vi "SetAllPulsersGUI.vi"(7 "Init Tabor?":bool=TRUE, 8 "Tabor handle in":refnum<k15>, 11 "Pulser":T1) -> ()   [LabVIEW 2022 SP3]
uses:
  pulser.ctl
  PulserGlobals.vi
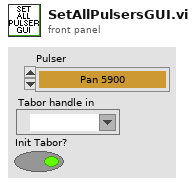
[diagram p1: front panel]
types:
  T1 = typedef "pulser.ctl" = enum16{"Pan 5900", "Daxsonics", "Agilent 33xxx", "UTEX", "JSR", "WMC Mono-Cycle", "No Pulser", "NYU AVTECH", "Tabor W1281A", "Pan 5800", "Unlisted", "Tabor WX2182B"}
  T2 = typedef "Daxsonics_Pulsers.ctl" = enum16{"BP1", "BP2_A", "BP2_B", "10ERS8", "New2021"}
  T3 = typedef "JSR Complete.ctl" = cluster{"JSR Pulse Settings":T4, "JSR Receive Settings":T9, "JSR Trigger Settings":T14}
  T4 = typedef "JSR Pulse.ctl" = cluster{"Damping":T5, "Pulse Energy Level":T6, "Pulser Impedance":T7, "Pulser Voltage (V)":T8}
  T5 = typedef "Damping.ctl" = i16
  T6 = typedef "Energy.ctl" = u16
  T7 = typedef "Z.ctl" = u16
  T8 = typedef "Volt.ctl" = i16
  T9 = typedef "JSR Recieve.ctl" = cluster{"Receiver Mode":T10, "High Pass Filter":T11, "Low Pass Filter":T12, "Gain (dB)":T13}
  T10 = typedef "Mode.ctl" = i8
  T11 = typedef "HPF.ctl" = u16
  T12 = typedef "LPF.ctl" = u16
  T13 = typedef "Gain.ctl" = i8
  T14 = typedef "JSR Trigger.ctl" = cluster{"External Trigger Limit":T15, "Trigger Source":T16, "PRF (Hz)":T17}
  T15 = typedef "Trig Limit.ctl" = i8
  T16 = typedef "Trig Source.ctl" = i8
  T17 = typedef "PRF.ctl" = dbl
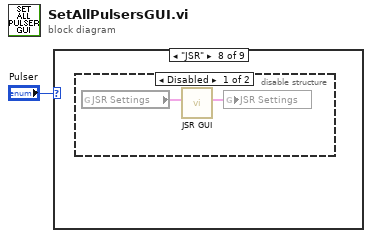
[diagram p0: block diagram]
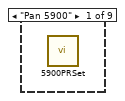
[diagram p2: hidden frame]
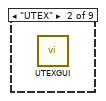
[diagram p3: hidden frame]
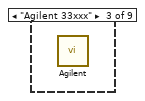
[diagram p4: hidden frame]
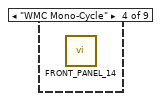
[diagram p5: hidden frame]
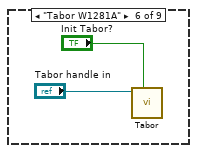
[diagram p7: hidden frame]
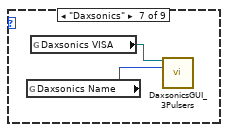
[diagram p8: hidden frame]
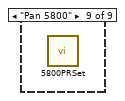
[diagram p10: hidden frame]
diagram:
  n1 = case shown="\"JSR\"" "Pulser" {
    frame "Pan 5900" {
      n2 = call "5900PRSet.vi"() -> ()  [unwired: 1 in, 15 out]
    }
    frame "UTEX" {
      n3 = call "UTEXGUI.vi"() -> ()  [unwired: 12 in]
    }
    frame "Agilent 33xxx" {
      n4 = call "Agilent.vi"() -> ()  [unwired: 12 out]
    }
    frame "WMC Mono-Cycle" {
      n5 = call "FRONT_PANEL_14.vi"() -> ()  [unwired: 16 out]
    }
    frame "No Pulser", Default {
    }
    frame "Tabor W1281A" {
      n6 = call "Tabor.vi"("Init?"="Init Tabor?", "Tabor handle in"="Tabor handle in") -> ()  [unwired: 8 in, 2 out]
    }
    frame "Daxsonics" {
      n7 = global read "PulserGlobals.vi" "Daxsonics Name"() -> (w4:T2)
      n8 = global read "PulserGlobals.vi" "Daxsonics VISA"() -> (w5:refnum<visa-resource-name>)
      n9 = call "DaxsonicsGUI_3Pulsers.vi"("Daxsonics VISA"=w5, "Daxsonics Name"=w4) -> ()  [unwired: 14 in]
    }
    frame "JSR" {
      n10 = disable-structure shown="Disabled" {
        frame Disabled {
          n11 = global read "PulserGlobals.vi" "JSR Settings"() -> (w7:T3)
          n12 = call "JSR GUI.vi"("JSR Complete"=w7) -> ("JSR Complete Out"=w6:T3)  [unwired: 8 in, 2 out]
          n13 = global write "PulserGlobals.vi" "JSR Settings"(w6) -> ()
        }
        frame Enabled {
        }
      }
    }
    frame "Pan 5800" {
      n14 = call "5800PRSet.vi"() -> ()  [unwired: 16 in]
    }
  }
